vi "nested_cluster_fields.vi"(10 "replacement":dbl, 11 "cluster_in":T1) -> (2 "original_right":dbl, 3 "cluster_out":T1)   [LabVIEW 2020]
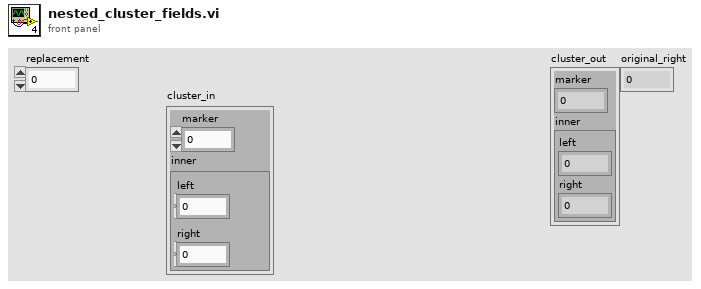
[diagram p1: front panel]
types:
  T1 = cluster{"marker":dbl, "inner":cluster{"left":dbl, "right":dbl}}
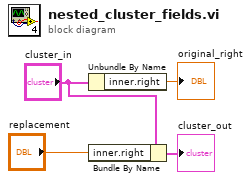
[diagram p0: block diagram]
diagram:
  n1 = Unbundle By Name("cluster_in") -> ("inner.right"=→"original_right":dbl)
  n2 = Bundle By Name(cluster="cluster_in", "inner.right"="replacement") -> (→"cluster_out":T1)
